vi "题目7.vi"() -> ()   [LabVIEW 2017]
uses:
  <vilib>/Utility/file.llb/Write Delimited Spreadsheet (DBL).vi
  <vilib>/measure/NI_MABase.lvlib
panel:
  out "数组":dbl[](array[numeric])
  out "波形图":waveform(dbl)(graph)
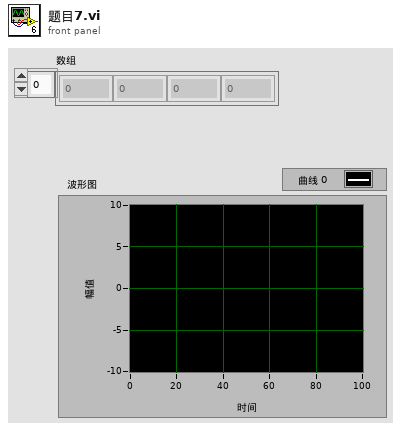
[diagram p1: front panel]
types:
  T1 = enum16{"open", "replace", "create", "open or create", "replace or create", "replace or create with confirmation"}
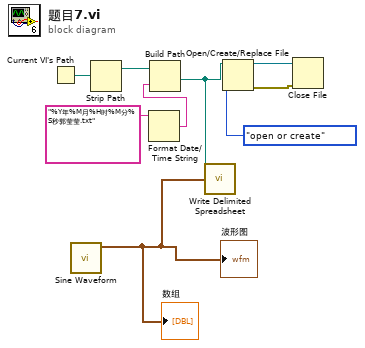
[diagram p0: block diagram]
diagram:
  n1 = Current VI's Path() -> (path=w9:path)
  n2 = call <vilib>:"Sine Waveform.vi"() -> ("signal out"=w1:waveform(dbl))  [unwired: 10 in, 1 out]
  "波形图" <- w1
  "数组" <- w1
  n3 = Strip Path(path=w9) -> (stripped path=w8:path)  [unwired: 1 out]
  n4 = Format Date/Time String(time format string (%c)="%Y年%M月%H时%M分%S秒郭莹莹.txt" ("时间格式字符串(%c)")) -> (date/time string=w7:string)  [unwired: 2 in]
  n5 = Build Path(base path=w8, name or relative path=w7) -> (appended path=w2:path)
  n6 = call-poly <vilib>:"Write Delimited Spreadsheet.vi"("file path (dialog if empty)"=w2, "1D data"=w1) -> ()  [unwired: 12 in, 2 out]
  n7 = Open/Create/Replace File(file path (use dialog)=w2, operation (0:open)=T1."open or create" ("操作(0:open)")) -> (refnum out=w5:refnum<file>, error out=w4:errorcluster)  [unwired: 4 in, 1 out]
  n8 = Close File(refnum=w5, error in=w4) -> ()  [unwired: 2 out]
